vi "Autonomous Independent.vi"   [LabVIEW 2015]
doc: "This VI is called when autonomous begins, and will automatically be terminated when autonomous ends. You can carry out timed or sensor driven robot movement independently without needing to return to the caller."
uses:
  <vilib>/Rock Robotics/Network Tables/NT Read Number.vi
panel:
  # "Be sure to right-click and choose Data Operations>>Make Current Value default if you want to save the array values with the VI"
types:
  T1 = typedef "WPI_MotorControlDeviceRef.ctl" = cluster{"DeviceStatus":errorcluster, "Type":T2, "PWM":cluster{"PWM Channel":T3, "DeadBand":T4}, "CAN":cluster{"Device Number":u8, "Control Mode":T5, "Semaphore":T6, "Max Vout":dbl, "TalonSRX Control Mode":T7}, "Invert":bool}
  T2 = typedef "WPI_MotorControlType.ctl" = enum16{"PWM", "CAN", "CANTalonSRX"}
  T3 = typedef "FPGA_DIOPWMChannel.ctl" = enum8{"PWM 0", "PWM 1", "PWM 2", "PWM 3", "PWM 4", "PWM 5", "PWM 6", "PWM 7", "PWM 8", "PWM 9", "PWM MXP 0", "PWM MXP 1", "PWM MXP 2", "PWM MXP 3", "PWM MXP 4", "PWM MXP 5", "PWM MXP 6", "PWM MXP 7", "PWM MXP 8", "PWM MXP 9", "Invalid"}
  T4 = typedef "WPI_PWMDeadband.ctl" = cluster{"Name":string, "maxPositivePwm":i32, "minPositivePwm":i32, "centerPwm":i32, "maxNegativePwm":i32, "minNegativePwm":i32, "angularRange":u16}
  T5 = typedef "WPI_CANJaguar_ControlMode.ctl" = enum8{"Percent VBus", "Current", "Speed", "Position", "Voltage"}
  T6 = typedef "Semaphore RefNum" = refnum<k1>
  T7 = typedef "WPI_CANTalonSRX_APIControlMode.ctl" = enum8{"Percent VBus", "Speed", "Position", "Slave", "Unchanged / Invalid", "Voltage Compensation", "Current", "Motion Profile"}
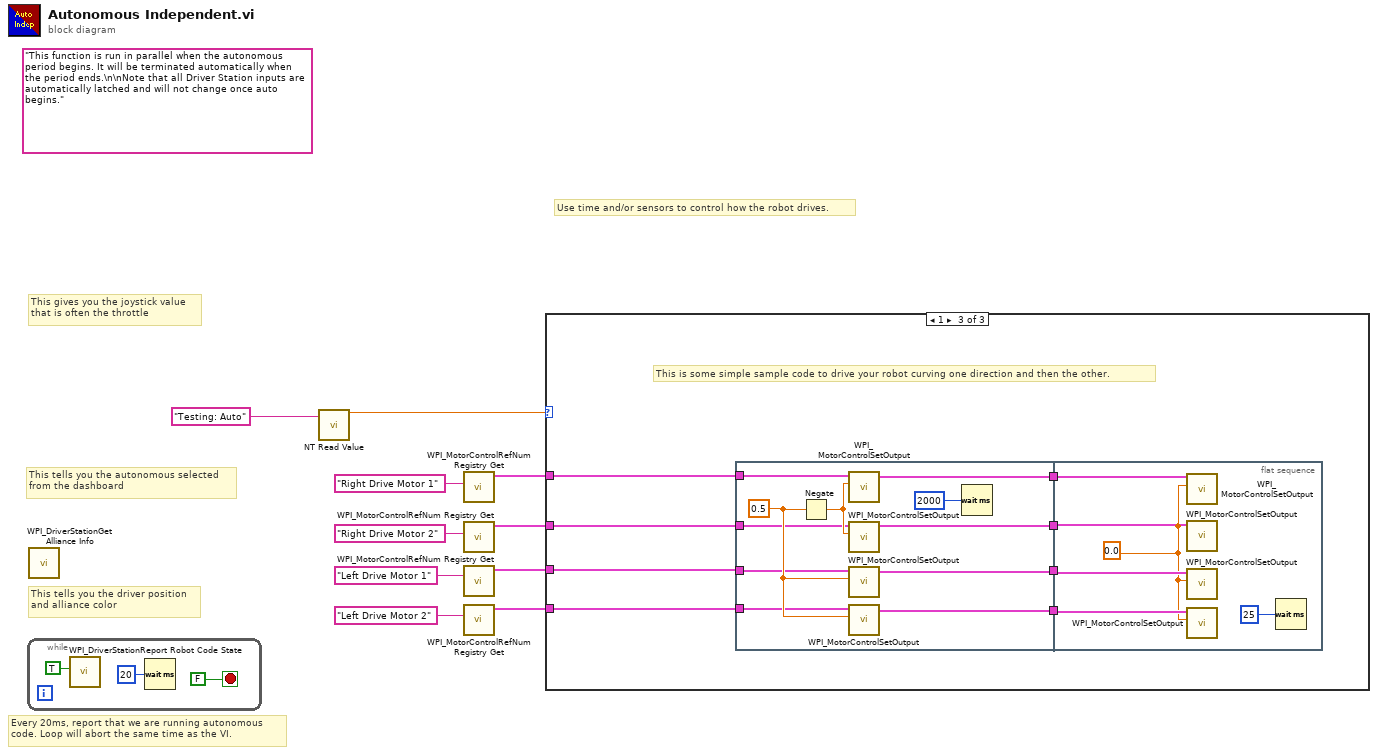
[diagram p0: block diagram]
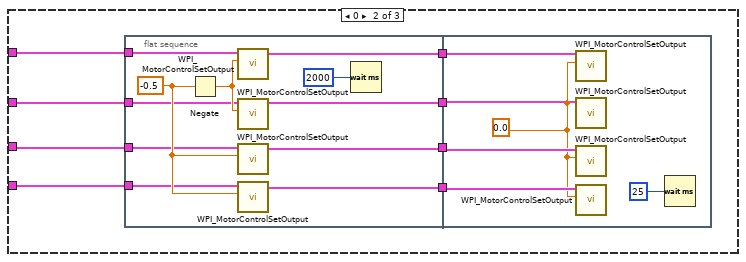
[diagram p3: hidden frame]
diagram:
  (unwired) "This function is run in parallel when the autonomous period begins. It will be terminated automatically when the period ends.\n\nNote that all Driver Station inputs are automatically latched and will not change once auto begins."
  # "This tells you the autonomous selected\nfrom the dashboard"
  # "Every 20ms, report that we are running autonomous\ncode. Loop will abort the same time as the VI."
  # "This gives you the joystick value\nthat is often the throttle"
  # "Use time and/or sensors to control how the robot drives."
  # "This tells you the driver position\nand alliance color"
  n1 = while {
    stop <- FALSE stop-if-true
    n2 = call <vilib>:"WPI_DriverStationReport Robot Code State.vi"("Autonomous"=TRUE) -> ()  [unwired: 10 in, 1 out]
    n3 = Wait (ms)(milliseconds to wait=u32 20) -> ()  [unwired: 1 out]
  }
  n4 = call <vilib>:"WPI_DriverStationGet Alliance Info.vi"() -> ()  [unwired: 12 out]
  n5 = call-poly <vilib>:"NT Read Value.vi"("Name"="Testing: Auto") -> ("Numeric"=w9:dbl)  [unwired: 9 in, 1 out]
  n6 = call <vilib>:"WPI_MotorControlRefNum Registry Get.vi"("refnum name"="Right Drive Motor 1") -> ("MotorControlDevRef"=w8:T1)  [unwired: 9 in, 1 out]
  n7 = call <vilib>:"WPI_MotorControlRefNum Registry Get.vi"("refnum name"="Right Drive Motor 2") -> ("MotorControlDevRef"=w7:T1)  [unwired: 9 in, 1 out]
  n8 = call <vilib>:"WPI_MotorControlRefNum Registry Get.vi"("refnum name"="Left Drive Motor 1") -> ("MotorControlDevRef"=w6:T1)  [unwired: 9 in, 1 out]
  n9 = call <vilib>:"WPI_MotorControlRefNum Registry Get.vi"("refnum name"="Left Drive Motor 2") -> ("MotorControlDevRef"=w5:T1)  [unwired: 9 in, 1 out]
  n10 = case shown="1" w9 {
    tunnel: w8 -> [_ w17 w39]
    tunnel: w7 -> [_ w16 w40]
    tunnel: w6 -> [_ w15 w41]
    tunnel: w5 -> [_ w14 w42]
    frame Default {
      # "You can put your main auto here, or you can right-click on the case and make any\nother frame be the default case."
      # "This is the frame that will execute if no selection is made, or if it is not recognized"
    }
    frame 0 {
      n11 = flat-sequence {
        tunnel: [w30] -> w21
        tunnel: [w29] -> w20
        tunnel: [w27] -> w19
        tunnel: [w28] -> w18
        tunnel: w17 -> [w25]
        tunnel: w16 -> [w24]
        tunnel: w15 -> [w23]
        tunnel: w14 -> [w22]
        tunnel: w21 -> [w38]
        tunnel: w20 -> [w37]
        tunnel: w19 -> [w36]
        tunnel: w18 -> [w35]
        frame #0 {
          w32 = -0.5
          n12 = Negate(x=w32) -> (-x=w31:dbl)
          n13 = call <vilib>:"WPI_MotorControlSetOutput.vi"("Output"=w31, "MotorControlDevRef"=w25) -> ("MotorControlDevRef"=w30:T1)  [unwired: 7 in, 2 out]
          n14 = call <vilib>:"WPI_MotorControlSetOutput.vi"("Output"=w31, "MotorControlDevRef"=w24) -> ("MotorControlDevRef"=w29:T1)  [unwired: 7 in, 2 out]
          n15 = call <vilib>:"WPI_MotorControlSetOutput.vi"("Output"=w32, "MotorControlDevRef"=w23) -> ("MotorControlDevRef"=w27:T1)  [unwired: 7 in, 2 out]
          n16 = call <vilib>:"WPI_MotorControlSetOutput.vi"("Output"=w32, "MotorControlDevRef"=w22) -> ("MotorControlDevRef"=w28:T1)  [unwired: 7 in, 2 out]
          n17 = Wait (ms)(milliseconds to wait=u32 2000) -> ()  [unwired: 1 out]
        }
        frame #1 {
          w34 = 0.0
          n18 = call <vilib>:"WPI_MotorControlSetOutput.vi"("Output"=w34, "MotorControlDevRef"=w38) -> ()  [unwired: 7 in, 3 out]
          n19 = call <vilib>:"WPI_MotorControlSetOutput.vi"("Output"=w34, "MotorControlDevRef"=w37) -> ()  [unwired: 7 in, 3 out]
          n20 = call <vilib>:"WPI_MotorControlSetOutput.vi"("Output"=w34, "MotorControlDevRef"=w36) -> ()  [unwired: 7 in, 3 out]
          n21 = call <vilib>:"WPI_MotorControlSetOutput.vi"("Output"=w34, "MotorControlDevRef"=w35) -> ()  [unwired: 7 in, 3 out]
          n22 = Wait (ms)(milliseconds to wait=u32 25) -> ()  [unwired: 1 out]
        }
      }
    }
    frame 1 {
      # "This is some simple sample code to drive your robot curving one direction and then the other."
      n23 = flat-sequence {
        tunnel: [w55] -> w46
        tunnel: [w54] -> w45
        tunnel: [w52] -> w44
        tunnel: [w53] -> w43
        tunnel: w39 -> [w50]
        tunnel: w40 -> [w49]
        tunnel: w41 -> [w48]
        tunnel: w42 -> [w47]
        tunnel: w46 -> [w63]
        tunnel: w45 -> [w62]
        tunnel: w44 -> [w61]
        tunnel: w43 -> [w60]
        frame #0 {
          w57 = 0.5
          n24 = Negate(x=w57) -> (-x=w56:dbl)
          n25 = call <vilib>:"WPI_MotorControlSetOutput.vi"("Output"=w56, "MotorControlDevRef"=w50) -> ("MotorControlDevRef"=w55:T1)  [unwired: 7 in, 2 out]
          n26 = call <vilib>:"WPI_MotorControlSetOutput.vi"("Output"=w56, "MotorControlDevRef"=w49) -> ("MotorControlDevRef"=w54:T1)  [unwired: 7 in, 2 out]
          n27 = call <vilib>:"WPI_MotorControlSetOutput.vi"("Output"=w57, "MotorControlDevRef"=w48) -> ("MotorControlDevRef"=w52:T1)  [unwired: 7 in, 2 out]
          n28 = call <vilib>:"WPI_MotorControlSetOutput.vi"("Output"=w57, "MotorControlDevRef"=w47) -> ("MotorControlDevRef"=w53:T1)  [unwired: 7 in, 2 out]
          n29 = Wait (ms)(milliseconds to wait=u32 2000) -> ()  [unwired: 1 out]
        }
        frame #1 {
          w59 = 0.0
          n30 = call <vilib>:"WPI_MotorControlSetOutput.vi"("Output"=w59, "MotorControlDevRef"=w63) -> ()  [unwired: 7 in, 3 out]
          n31 = call <vilib>:"WPI_MotorControlSetOutput.vi"("Output"=w59, "MotorControlDevRef"=w62) -> ()  [unwired: 7 in, 3 out]
          n32 = call <vilib>:"WPI_MotorControlSetOutput.vi"("Output"=w59, "MotorControlDevRef"=w61) -> ()  [unwired: 7 in, 3 out]
          n33 = call <vilib>:"WPI_MotorControlSetOutput.vi"("Output"=w59, "MotorControlDevRef"=w60) -> ()  [unwired: 7 in, 3 out]
          n34 = Wait (ms)(milliseconds to wait=u32 25) -> ()  [unwired: 1 out]
        }
      }
    }
  }
